vi "SDG60ConfArbWaveform1new.vi"(0 "VISA resource name":refnum<visa-resource-name>="USB0::0xF4EC::0x1101::SDG6XEBC5R0119::INSTR", 1 "Freq/SR/P (1 Hz)":dbl=1.0 min=1e-06 max=160000000.0 step=1.0 format="%#.15g", 2 "DDS/TArb 0: DDS":i32(ring)=1 items=["DDS", "TrueArb"], 5 "Select Channel (1:Channel 1)":i32(ring)=1 items=["Channel 1"=1, "Channel 2"=2], 7 "Amplitude(0.1 Vpp)":dbl=0.1 min=0.001 max=20.0 step=1.0 format="%#.15f", 9 "Offset (0.00 V)":dbl min=-10.0 max=10.0 format="%#_15g", 11 "error in (no error)":errorcluster, 12 "Select Freq/SR/P (0:Freq)":i32(ring) items=["Frequency", "Sample Rate", "Period"], 13 "Interpolation 0: Zero-order":i32(ring) items=["Zero-Order", "Linear", "Sinc", "Sin27", "Sinc13"]) -> (4 "VISA resource name out":refnum<visa-resource-name>, 15 "error out":errorcluster)   [LabVIEW 2018]
doc: "Sets the waveform parameters for an arbitrary waveform. This VI should be called after <b>Create Arbitrary Waveform.vi</b> (for user defined arbitrary waveform) and <b>Select Arbitrary Waveform.vi</b>"
panel:
  in  "Phase (0 deg)":dbl min=-360.0 max=360.0 format="%#.15g"
  # "Must precede with SDG60SelectArbitraryWFM\nMay take time (~20s) if WFM is large"
  # "Sinc type interpolations use virtual keys\nVirtual keys not used for zero-hold & linear\nInterpolation method, is only for TrueArb"
  # "Range: 2mVpp-20Vpp. \n6 digits precision"
  # "Range: -10V-10V\n6 digits precision"
  # "Freq (DDS): 1uHz-50MHz \nFreq (TrueArb): 1uHz- Max depends on WFM length\nSR: 1uS/s-300MSa/s\nP: 20ns-1Ms\n10 Digit precision for F & SR\n6 Digit precision for P"
  # "For TrueArb use only F or SR \nFor DDS use F or P\nMay take time (few seconds!) to switch to TrueArb if WFM is large"
  # "Range -360..360deg, larger values will be warped. Resolution 0.0001 deg"
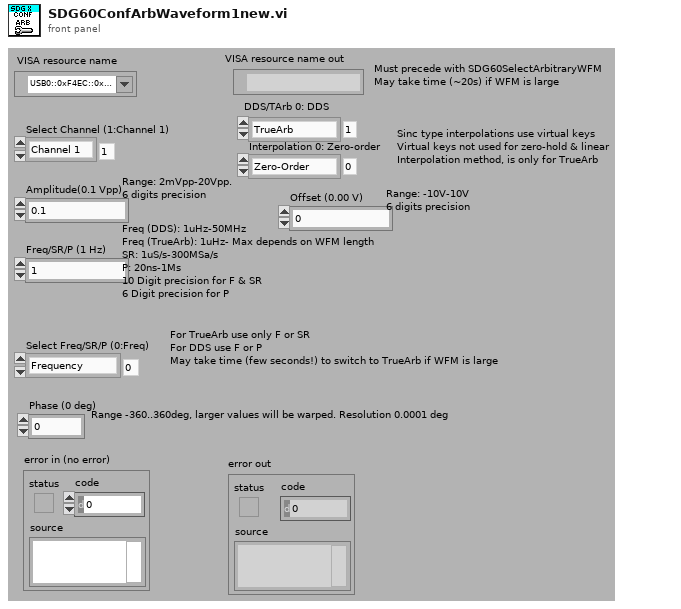
[diagram p1: front panel]
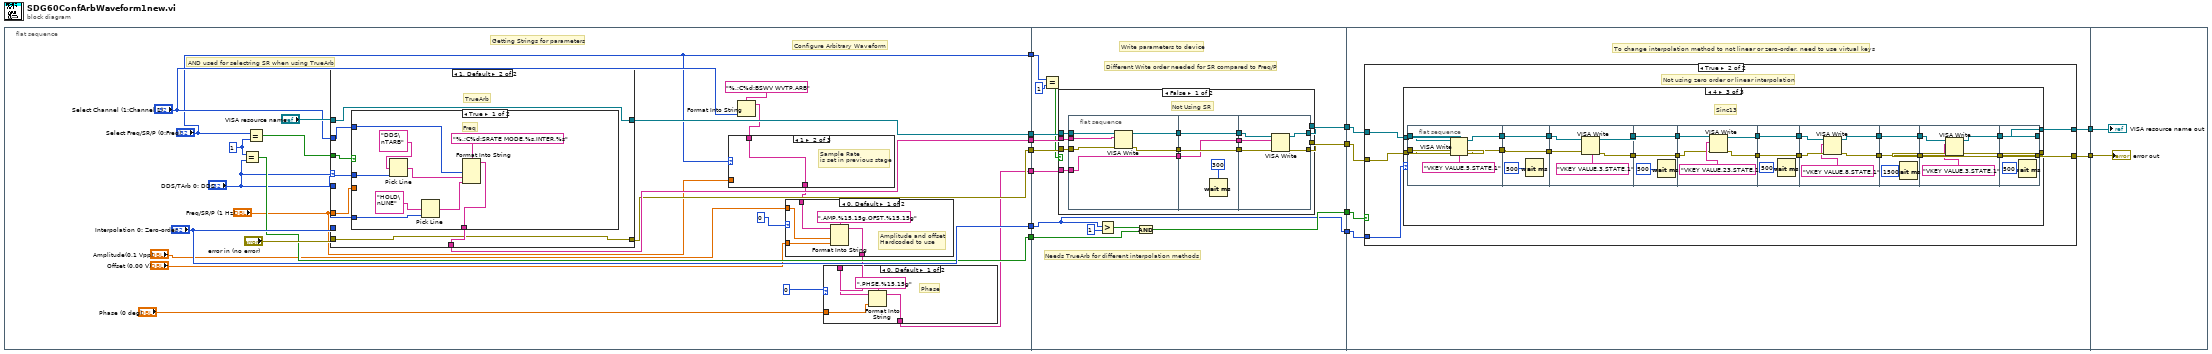
[diagram p0: block diagram]
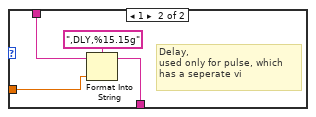
[diagram p2: hidden frame]
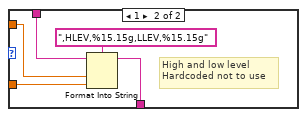
[diagram p3: hidden frame]
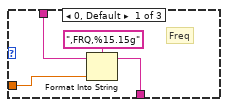
[diagram p4: hidden frame]
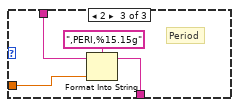
[diagram p5: hidden frame]
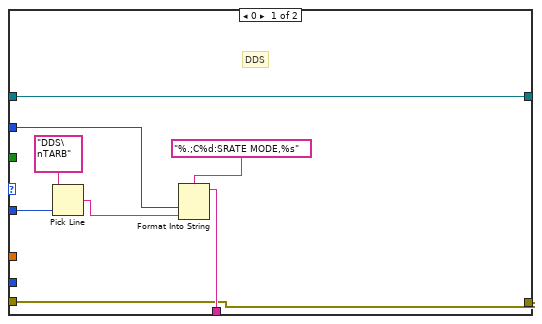
[diagram p6: hidden frame]
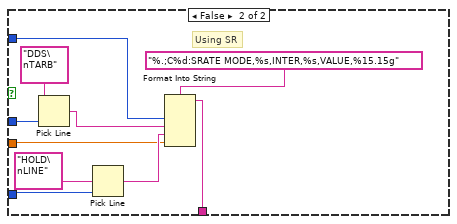
[diagram p7: hidden frame]
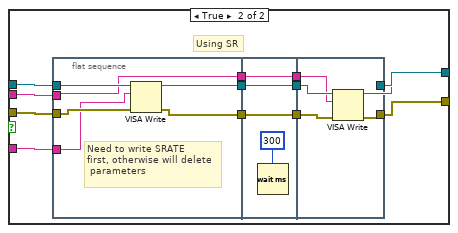
[diagram p8: hidden frame]
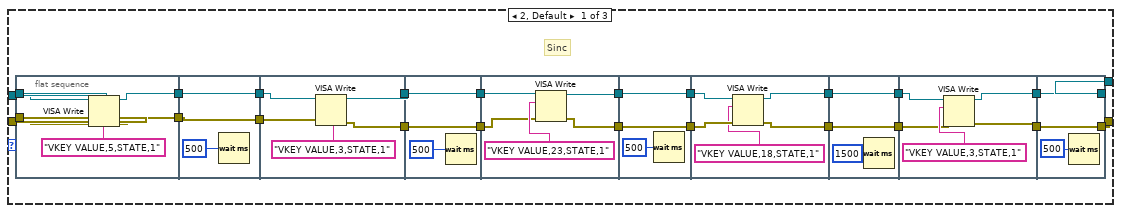
[diagram p10: hidden frame]
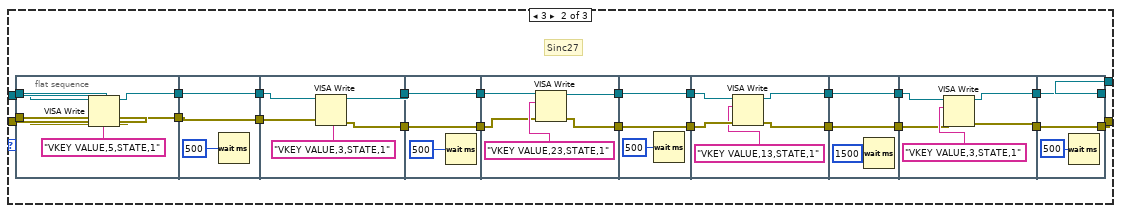
[diagram p11: hidden frame]
diagram:
  n1 = flat-sequence {
    tunnel: [w34] -> w13
    tunnel: [w19] -> w12
    tunnel: [w33] -> w11
    tunnel: [w32] -> w10
    tunnel: [w30] -> w9
    tunnel: ["Interpolation 0: Zero-order"] -> w8
    tunnel: ["Select Freq/SR/P (0:Freq)"] -> w1
    tunnel: w13 -> [w112]
    tunnel: w12 -> [w111]
    tunnel: w11 -> [w110]
    tunnel: w10 -> [w109]
    tunnel: w9 -> [w105]
    tunnel: w8 -> [w102]
    tunnel: [w108] -> w7
    tunnel: [w107] -> w6
    tunnel: [w104] -> w5
    tunnel: [w102] -> w4
    tunnel: w1 -> [w100]
    tunnel: w7 -> [w171]
    tunnel: w6 -> [w170]
    tunnel: w5 -> [w172]
    tunnel: w4 -> [w169]
    tunnel: [w168] -> w3
    tunnel: [w167] -> w2
    tunnel: w3 -> [w366]
    tunnel: w2 -> [w367]
    frame #0 {
      w29 = 1
      # "Getting Strings for parameters"
      # "AND used for selectring SR when using TrueArb"
      # "Configure Arbitrary Waveform"
      n2 = Equal?(x=w29, y="DDS/TArb 0: DDS") -> (x = y?=w30:bool)
      n3 = Equal?(x="Select Freq/SR/P (0:Freq)", y=w29) -> (x = y?=w14:bool)
      n4 = case shown="1, Default" "DDS/TArb 0: DDS" {
        tunnel: "Interpolation 0: Zero-order" -> [_ w79]
        tunnel: "DDS/TArb 0: DDS" -> [w70 w78]
        tunnel: "Select Channel (1:Channel 1)" -> [w68 w77]
        tunnel: [w67 w76] -> w34
        tunnel: w14 -> [_ w72]
        tunnel: "VISA resource name" -> [w65 w75]
        tunnel: "error in (no error)" -> [w64 w74]
        tunnel: [w65 w75] -> w32
        tunnel: [w64 w74] -> w33
        tunnel: "Freq/SR/P (1 Hz)" -> [_ w73]
        frame 0 {
          # "DDS"
          n5 = Pick Line(multi-line string="DDS\nTARB", line index=w70) -> (output string=w69:string)  [unwired: 1 in]
          n6 = Format Into String(format string="%.;C%d:SRATE MODE,%s", w68, w69) -> (resulting string=w67:string)  [unwired: 2 in, 1 out]
        }
        frame 1, Default {
          # "TrueArb"
          n7 = case shown="True" w72 {
            tunnel: w79 -> [w80 w97]
            tunnel: w78 -> [w82 w95]
            tunnel: w77 -> [w83 w93]
            tunnel: [w81 w92] -> w76
            tunnel: w73 -> [_ w89]
            frame True {
              # "Freq"
              n8 = Pick Line(multi-line string="DDS\nTARB", line index=w82) -> (output string=w88:string)  [unwired: 1 in]
              n9 = Pick Line(multi-line string="HOLD\nLINE", line index=w80) -> (output string=w87:string)  [unwired: 1 in]
              n10 = Format Into String(format string="%.;C%d:SRATE MODE,%s,INTER,%s", w83, w88, w87) -> (resulting string=w81:string)  [unwired: 2 in, 1 out]
            }
            frame False {
              # "Using SR"
              n11 = Pick Line(multi-line string="DDS\nTARB", line index=w95) -> (output string=w94:string)  [unwired: 1 in]
              n12 = Pick Line(multi-line string="HOLD\nLINE", line index=w97) -> (output string=w96:string)  [unwired: 1 in]
              n13 = Format Into String(format string="%.;C%d:SRATE MODE,%s,INTER,%s,VALUE,%15.15g", w93, w94, w96, w89) -> (resulting string=w92:string)  [unwired: 2 in, 1 out]
            }
          }
        }
      }
      n14 = Format Into String(format string="%.;C%d:BSWV WVTP,ARB", "Select Channel (1:Channel 1)") -> (resulting string=w27:string)  [unwired: 2 in, 1 out]
      n15 = case shown="1" "Select Freq/SR/P (0:Freq)" {
        tunnel: w27 -> [w58 w59 w63]
        tunnel: [w56 w59 w61] -> w20
        tunnel: "Freq/SR/P (1 Hz)" -> [w55 _ w60]
        frame 0, Default {
          # "Freq"
          n16 = Format Into String(format string=",FRQ,%15.15g", initial string=w58, w55) -> (resulting string=w56:string)  [unwired: 1 in, 1 out]
        }
        frame 1 {
          # "Sample Rate\nis set in previous stage"
        }
        frame 2 {
          # "Period"
          n17 = Format Into String(format string=",PERI,%15.15g", initial string=w63, w60) -> (resulting string=w61:string)  [unwired: 1 in, 1 out]
        }
      }
      n18 = case shown="0, Default" 0 {
        tunnel: [w48 w53] -> w18
        tunnel: "Amplitude(0.1 Vpp)" -> [w47 w52]
        tunnel: "Offset (0.00 V)" -> [w46 w51]
        tunnel: w20 -> [w45 w50]
        frame 0, Default {
          # "Amplitude and offset\nHardcoded to use"
          n19 = Format Into String(format string=",AMP,%15.15g,OFST,%15.15g", initial string=w45, w47, w46) -> (resulting string=w48:string)  [unwired: 1 in, 1 out]
        }
        frame 1 {
          # "High and low level\nHardcoded not to use"
          n20 = Format Into String(format string=",HLEV,%15.15g,LLEV,%15.15g", initial string=w50, w52, w51) -> (resulting string=w53:string)  [unwired: 1 in, 1 out]
        }
      }
      n21 = case shown="0, Default" 0 {
        tunnel: [w39 w43] -> w19
        tunnel: w18 -> [w38 w42]
        tunnel: "Phase (0 deg)" -> [w37 w41]
        frame 0, Default {
          # "Phase"
          n22 = Format Into String(format string=",PHSE,%15.15g", initial string=w38, w37) -> (resulting string=w39:string)  [unwired: 1 in, 1 out]
        }
        frame 1 {
          # "Delay,\nused only for pulse, which \nhas a seperate vi"
          n23 = Format Into String(format string=",DLY,%15.15g", initial string=w42, w41) -> (resulting string=w43:string)  [unwired: 1 in, 1 out]
        }
      }
    }
    frame #1 {
      # "Different Write order needed for SR compared to Freq/P"
      # "Write parameters to device"
      # "Needs TrueArb for different interpolation methods"
      n24 = Equal?(x=w100, y=1) -> (x = y?=w99:bool)
      n25 = case shown="False" w99 {
        tunnel: w112 -> [w118 w147]
        tunnel: w111 -> [w117 w146]
        tunnel: w110 -> [w116 w145]
        tunnel: w109 -> [w115 w144]
        tunnel: [w114 w143] -> w108
        tunnel: [w113 w142] -> w107
        frame False {
          # "Not Using SR"
          n26 = flat-sequence {
            tunnel: [w129] -> w124
            tunnel: w118 -> [w130]
            tunnel: [w128] -> w123
            tunnel: w117 -> [w127]
            tunnel: [w127] -> w122
            tunnel: w116 -> [w126]
            tunnel: w115 -> [w125]
            tunnel: w124 -> [w133]
            tunnel: [w133] -> w121
            tunnel: [w132] -> w120
            tunnel: w123 -> [w132]
            tunnel: w122 -> [w131]
            tunnel: [w131] -> w119
            tunnel: [w135] -> w114
            tunnel: w121 -> [w136]
            tunnel: w120 -> [w139]
            tunnel: [w138] -> w113
            tunnel: w119 -> [w137]
            frame #0 {
              n27 = VISA Write(VISA resource name=w125, write buffer=w130, error in (no error)=w126) -> (VISA resource name out=w129:refnum<visa-resource-name>, error out=w128:errorcluster)  [unwired: 1 out]
            }
            frame #1 {
              n28 = Wait (ms)(milliseconds to wait=300 ("x")) -> ()  [unwired: 1 out]
            }
            frame #2 {
              n29 = VISA Write(VISA resource name=w136, write buffer=w137, error in (no error)=w139) -> (VISA resource name out=w135:refnum<visa-resource-name>, error out=w138:errorcluster)  [unwired: 1 out]
            }
          }
        }
        frame True {
          # "Using SR"
          n30 = flat-sequence {
            tunnel: [w157] -> w151
            tunnel: w147 -> [w153]
            tunnel: [w156] -> w150
            tunnel: w146 -> [w152]
            tunnel: w145 -> [w155]
            tunnel: w144 -> [w154]
            tunnel: [w153] -> w140
            tunnel: w151 -> [w160]
            tunnel: [w160] -> w149
            tunnel: [w159] -> w148
            tunnel: w150 -> [w159]
            tunnel: [w158] -> w141
            tunnel: w140 -> [w158]
            tunnel: [w163] -> w143
            tunnel: w149 -> [w164]
            tunnel: w148 -> [w166]
            tunnel: [w165] -> w142
            tunnel: w141 -> [w162]
            frame #0 {
              # "Need to write SRATE\nfirst, otherwise will delete\n parameters"
              n31 = VISA Write(VISA resource name=w154, write buffer=w152, error in (no error)=w155) -> (VISA resource name out=w157:refnum<visa-resource-name>, error out=w156:errorcluster)  [unwired: 1 out]
            }
            frame #1 {
              n32 = Wait (ms)(milliseconds to wait=300 ("x")) -> ()  [unwired: 1 out]
            }
            frame #2 {
              n33 = VISA Write(VISA resource name=w164, write buffer=w162, error in (no error)=w166) -> (VISA resource name out=w163:refnum<visa-resource-name>, error out=w165:errorcluster)  [unwired: 1 out]
            }
          }
        }
      }
      n34 = Greater?(x=w102, y=1) -> (0:w106:bool)
      n35 = And(x=w106, y=w105) -> (x .and. y?=w104:bool)
    }
    frame #2 {
      # "To change interpolation method to not linear or zero-order, need to use virtual keys"
      n36 = case shown="True" w172 {
        tunnel: [w174 w175] -> w168
        tunnel: [w173 w176] -> w167
        tunnel: w171 -> [w174 w178]
        tunnel: w170 -> [w173 w177]
        tunnel: w169 -> [_ w179]
        frame False {
          # "Using Zero order or linear interpolation"
        }
        frame True {
          # "Not using zero order or linear interpolation"
          n37 = case shown="4" w179 {
            tunnel: w178 -> [w196 w258 w320]
            tunnel: w177 -> [w197 w259 w321]
            tunnel: [w194 w256 w318] -> w176
            tunnel: [w195 w257 w319] -> w175
            frame 2, Default {
              # "Sinc"
              n38 = flat-sequence {
                tunnel: w197 -> [w206]
                tunnel: w196 -> [w205]
                tunnel: [w204] -> w201
                tunnel: [w202] -> w200
                tunnel: w201 -> [w209]
                tunnel: [w209] -> w199
                tunnel: [w207] -> w198
                tunnel: w200 -> [w207]
                tunnel: w199 -> [w213]
                tunnel: w198 -> [w210]
                tunnel: [w212] -> w193
                tunnel: [w211] -> w192
                tunnel: w193 -> [w217]
                tunnel: [w217] -> w191
                tunnel: w192 -> [w216]
                tunnel: [w216] -> w189
                tunnel: w191 -> [w222]
                tunnel: [w218] -> w190
                tunnel: w189 -> [w220]
                tunnel: [w219] -> w188
                tunnel: w190 -> [w225]
                tunnel: w188 -> [w224]
                tunnel: [w225] -> w187
                tunnel: [w224] -> w186
                tunnel: w187 -> [w230]
                tunnel: w186 -> [w229]
                tunnel: [w227] -> w185
                tunnel: [w228] -> w184
                tunnel: w185 -> [w233]
                tunnel: w184 -> [w232]
                tunnel: [w233] -> w183
                tunnel: [w232] -> w182
                tunnel: w183 -> [w238]
                tunnel: w182 -> [w235]
                tunnel: [w237] -> w181
                tunnel: [w234] -> w180
                tunnel: [w240] -> w194
                tunnel: [w241] -> w195
                tunnel: w181 -> [w241]
                tunnel: w180 -> [w240]
                frame #0 {
                  n39 = VISA Write(VISA resource name=w205, write buffer="VKEY VALUE,5,STATE,1", error in (no error)=w206) -> (VISA resource name out=w204:refnum<visa-resource-name>, error out=w202:errorcluster)  [unwired: 1 out]
                }
                frame #1 {
                  n40 = Wait (ms)(milliseconds to wait=500) -> ()  [unwired: 1 out]
                }
                frame #2 {
                  n41 = VISA Write(VISA resource name=w213, write buffer="VKEY VALUE,3,STATE,1", error in (no error)=w210) -> (VISA resource name out=w212:refnum<visa-resource-name>, error out=w211:errorcluster)  [unwired: 1 out]
                }
                frame #3 {
                  n42 = Wait (ms)(milliseconds to wait=500) -> ()  [unwired: 1 out]
                }
                frame #4 {
                  n43 = VISA Write(VISA resource name=w222, write buffer="VKEY VALUE,23,STATE,1", error in (no error)=w220) -> (VISA resource name out=w218:refnum<visa-resource-name>, error out=w219:errorcluster)  [unwired: 1 out]
                }
                frame #5 {
                  n44 = Wait (ms)(milliseconds to wait=500) -> ()  [unwired: 1 out]
                }
                frame #6 {
                  n45 = VISA Write(VISA resource name=w230, write buffer="VKEY VALUE,18,STATE,1", error in (no error)=w229) -> (VISA resource name out=w227:refnum<visa-resource-name>, error out=w228:errorcluster)  [unwired: 1 out]
                }
                frame #7 {
                  n46 = Wait (ms)(milliseconds to wait=1500) -> ()  [unwired: 1 out]
                }
                frame #8 {
                  n47 = VISA Write(VISA resource name=w238, write buffer="VKEY VALUE,3,STATE,1", error in (no error)=w235) -> (VISA resource name out=w237:refnum<visa-resource-name>, error out=w234:errorcluster)  [unwired: 1 out]
                }
                frame #9 {
                  n48 = Wait (ms)(milliseconds to wait=500) -> ()  [unwired: 1 out]
                }
              }
            }
            frame 3 {
              # "Sinc27"
              n49 = flat-sequence {
                tunnel: w259 -> [w268]
                tunnel: w258 -> [w267]
                tunnel: [w266] -> w263
                tunnel: [w264] -> w262
                tunnel: w263 -> [w271]
                tunnel: [w271] -> w261
                tunnel: [w269] -> w260
                tunnel: w262 -> [w269]
                tunnel: w261 -> [w275]
                tunnel: w260 -> [w272]
                tunnel: [w274] -> w255
                tunnel: [w273] -> w254
                tunnel: w255 -> [w279]
                tunnel: [w279] -> w253
                tunnel: w254 -> [w278]
                tunnel: [w278] -> w251
                tunnel: w253 -> [w284]
                tunnel: [w280] -> w252
                tunnel: w251 -> [w282]
                tunnel: [w281] -> w250
                tunnel: w252 -> [w287]
                tunnel: w250 -> [w286]
                tunnel: [w287] -> w249
                tunnel: [w286] -> w248
                tunnel: w249 -> [w292]
                tunnel: w248 -> [w291]
                tunnel: [w289] -> w247
                tunnel: [w290] -> w246
                tunnel: w247 -> [w295]
                tunnel: w246 -> [w294]
                tunnel: [w295] -> w245
                tunnel: [w294] -> w244
                tunnel: w245 -> [w300]
                tunnel: w244 -> [w297]
                tunnel: [w299] -> w243
                tunnel: [w296] -> w242
                tunnel: [w302] -> w256
                tunnel: [w303] -> w257
                tunnel: w243 -> [w303]
                tunnel: w242 -> [w302]
                frame #0 {
                  n50 = VISA Write(VISA resource name=w267, write buffer="VKEY VALUE,5,STATE,1", error in (no error)=w268) -> (VISA resource name out=w266:refnum<visa-resource-name>, error out=w264:errorcluster)  [unwired: 1 out]
                }
                frame #1 {
                  n51 = Wait (ms)(milliseconds to wait=500) -> ()  [unwired: 1 out]
                }
                frame #2 {
                  n52 = VISA Write(VISA resource name=w275, write buffer="VKEY VALUE,3,STATE,1", error in (no error)=w272) -> (VISA resource name out=w274:refnum<visa-resource-name>, error out=w273:errorcluster)  [unwired: 1 out]
                }
                frame #3 {
                  n53 = Wait (ms)(milliseconds to wait=500) -> ()  [unwired: 1 out]
                }
                frame #4 {
                  n54 = VISA Write(VISA resource name=w284, write buffer="VKEY VALUE,23,STATE,1", error in (no error)=w282) -> (VISA resource name out=w280:refnum<visa-resource-name>, error out=w281:errorcluster)  [unwired: 1 out]
                }
                frame #5 {
                  n55 = Wait (ms)(milliseconds to wait=500) -> ()  [unwired: 1 out]
                }
                frame #6 {
                  n56 = VISA Write(VISA resource name=w292, write buffer="VKEY VALUE,13,STATE,1", error in (no error)=w291) -> (VISA resource name out=w289:refnum<visa-resource-name>, error out=w290:errorcluster)  [unwired: 1 out]
                }
                frame #7 {
                  n57 = Wait (ms)(milliseconds to wait=1500) -> ()  [unwired: 1 out]
                }
                frame #8 {
                  n58 = VISA Write(VISA resource name=w300, write buffer="VKEY VALUE,3,STATE,1", error in (no error)=w297) -> (VISA resource name out=w299:refnum<visa-resource-name>, error out=w296:errorcluster)  [unwired: 1 out]
                }
                frame #9 {
                  n59 = Wait (ms)(milliseconds to wait=500) -> ()  [unwired: 1 out]
                }
              }
            }
            frame 4 {
              # "Sinc13"
              n60 = flat-sequence {
                tunnel: w321 -> [w330]
                tunnel: w320 -> [w329]
                tunnel: [w328] -> w325
                tunnel: [w326] -> w324
                tunnel: w325 -> [w333]
                tunnel: [w333] -> w323
                tunnel: [w331] -> w322
                tunnel: w324 -> [w331]
                tunnel: w323 -> [w337]
                tunnel: w322 -> [w334]
                tunnel: [w336] -> w317
                tunnel: [w335] -> w316
                tunnel: w317 -> [w341]
                tunnel: [w341] -> w315
                tunnel: w316 -> [w340]
                tunnel: [w340] -> w313
                tunnel: w315 -> [w346]
                tunnel: [w342] -> w314
                tunnel: w313 -> [w344]
                tunnel: [w343] -> w312
                tunnel: w314 -> [w349]
                tunnel: w312 -> [w348]
                tunnel: [w349] -> w311
                tunnel: [w348] -> w310
                tunnel: w311 -> [w354]
                tunnel: w310 -> [w353]
                tunnel: [w351] -> w309
                tunnel: [w352] -> w308
                tunnel: w309 -> [w357]
                tunnel: w308 -> [w356]
                tunnel: [w357] -> w307
                tunnel: [w356] -> w306
                tunnel: w307 -> [w362]
                tunnel: w306 -> [w359]
                tunnel: [w361] -> w305
                tunnel: [w358] -> w304
                tunnel: [w364] -> w318
                tunnel: [w365] -> w319
                tunnel: w305 -> [w365]
                tunnel: w304 -> [w364]
                frame #0 {
                  n61 = VISA Write(VISA resource name=w329, write buffer="VKEY VALUE,5,STATE,1", error in (no error)=w330) -> (VISA resource name out=w328:refnum<visa-resource-name>, error out=w326:errorcluster)  [unwired: 1 out]
                }
                frame #1 {
                  n62 = Wait (ms)(milliseconds to wait=500) -> ()  [unwired: 1 out]
                }
                frame #2 {
                  n63 = VISA Write(VISA resource name=w337, write buffer="VKEY VALUE,3,STATE,1", error in (no error)=w334) -> (VISA resource name out=w336:refnum<visa-resource-name>, error out=w335:errorcluster)  [unwired: 1 out]
                }
                frame #3 {
                  n64 = Wait (ms)(milliseconds to wait=500) -> ()  [unwired: 1 out]
                }
                frame #4 {
                  n65 = VISA Write(VISA resource name=w346, write buffer="VKEY VALUE,23,STATE,1", error in (no error)=w344) -> (VISA resource name out=w342:refnum<visa-resource-name>, error out=w343:errorcluster)  [unwired: 1 out]
                }
                frame #5 {
                  n66 = Wait (ms)(milliseconds to wait=500) -> ()  [unwired: 1 out]
                }
                frame #6 {
                  n67 = VISA Write(VISA resource name=w354, write buffer="VKEY VALUE,8,STATE,1", error in (no error)=w353) -> (VISA resource name out=w351:refnum<visa-resource-name>, error out=w352:errorcluster)  [unwired: 1 out]
                }
                frame #7 {
                  n68 = Wait (ms)(milliseconds to wait=1500) -> ()  [unwired: 1 out]
                }
                frame #8 {
                  n69 = VISA Write(VISA resource name=w362, write buffer="VKEY VALUE,3,STATE,1", error in (no error)=w359) -> (VISA resource name out=w361:refnum<visa-resource-name>, error out=w358:errorcluster)  [unwired: 1 out]
                }
                frame #9 {
                  n70 = Wait (ms)(milliseconds to wait=500) -> ()  [unwired: 1 out]
                }
              }
            }
          }
        }
      }
    }
    frame #3 {
      "VISA resource name out" <- w366
      "error out" <- w367
    }
  }
